vi "HFRR ADV v05.vi"() -> ()   [LabVIEW 2025] (continued)
            n1468 = local write "yflag"(1.0 ("tflag")) -> ()
            n1469 = local write "zflag"(3.0 ("zflag")) -> ()
          }
        }
        n1470 = local read "acq 2"() -> (w2134:bool)
        n1471 = local read "AIR TEMP"() -> (w2097:dbl)
        n1472 = local read "Amb temp"() -> (w2101:dbl)
        n1473 = case shown="True" "Save & Continue" {
          frame False {
          }
          frame True {
            "acq 2" <- TRUE ("acq 2")
          }
        }
        n1474 = case shown="True" "Save & Continue" {
          frame False {
          }
          frame True {
            n1475 = while {
              tunnel: "0123456789abcdefghijklmnopqrstuvwxyzABCDEFGHIJKLMNOPQRSTUVWXYZ" ("string 2") -> [w2294]
              shift-right: [w2292] -> w2287
              shift-left: "" -> [w2291]
              i -> [w2301]
              stop <- w2300 stop-if-true
              n1476 = Random Number (0-1)() -> (number: 0 to 1=w2295:dbl)
              n1477 = Multiply(x=w2295, y=62.0) -> (x*y=w2297:dbl)
              n1478 = Decrement(x="Length") -> (x-1=w2290:i16)
              n1479 = To Word Integer(number=w2297) -> (16bit integer=w2298:i16)
              n1480 = String Subset(string=w2294, offset (0)=w2298, length (rest)=1 ("length (rest)")) -> (substring=w2293:string)
              n1481 = Greater Or Equal?(x=w2301, y=w2290) -> (x >= y?=w2300:bool)
              n1482 = Concatenate Strings(w2293, w2291) -> (w2292:string)
            }
            n1483 = local write "UUID"(w2287) -> ()
          }
        }
        n1484 = case shown="True" "Save & Continue" {
          frame False {
          }
          frame True {
            n1485 = local read "Operator ID"() -> (w2581:string)
            n1486 = local read "FILE"() -> (w2587:string)
            n1487 = String Length(string=w2587) -> (length=w2585:i32)
            n1488 = String Length(string=w2581) -> (length=w2582:i32)
            n1489 = Greater?(x=w2585, y=0) -> (0:w2584:bool)
            n1490 = Greater?(x=w2582, y=0) -> (0:w2580:bool)
            n1491 = And(x=w2584, y=w2580) -> (x .and. y?=w2579:bool)
            n1492 = case shown="True" w2579 {
              frame False {
                n1493 = stacked-sequence {
                  frame #0 {
                    n1494 = One Button Dialog(message="Please Enter a File Name and Operator ID to save data !", button name ("OK")="Ok") -> ()  [unwired: 1 out]
                  }
                  frame #1 {
                    n1495 = local write "Save & Continue"(FALSE ("OK Button")) -> ()
                  }
                }
                n1496 = local write "Save & Continue"(FALSE ("OK Button")) -> ()
              }
              frame True {
                n1497 = stacked-sequence {
                  frame #0 {
                    w2592 = 0.0
                    w2594 = cluster{"y":dbl, dbl, "y":dbl}[] [] ("History Data")
                    w2595 = FALSE ("Heater Button")
                    (unwired) ")!" ("string")
                    (unwired) ")" ("string")
                    w2593 = dbl[] [] ("History Data")
                    w2599 = "\r"
                    # "C:\\WinDucom\\Data\\"
                    # "C:\\LAB-IQ-NXT\\data"
                    n1498 = local write "Humidity ( %RH )"(w2592) -> ()
                    n1499 = local write "Frequency ( Hz )"(w2592) -> ()
                    n1500 = local write "speedop"(0.0 ("PIDclk 2")) -> ()
                    n1501 = local write "Set Temp 2"(w2592) -> ()
                    n1502 = local write "AIR TEMP"(w2592) -> ()
                    n1503 = local write "clk"(0.0 ("clk")) -> ()
                    n1504 = local write "Stroke 4"(w2592) -> ()
                    n1505 = local write "Stroke"(w2592) -> ()
                    n1506 = local write "COF 3"(w2592) -> ()
                    n1507 = local write "COF 2"(w2592) -> ()
                    n1508 = local write "TEMP"(w2592) -> ()
                    n1509 = local write "ecr 3"(w2592) -> ()
                    n1510 = local write "FF 3"(w2592) -> ()
                    n1511 = local write "FF 2"(w2592) -> ()
                    n1512 = property on="Humidity ( %RH )" class="WFChart (strict)"("History Data"=w2593) -> ()  [unwired: 2 in, 2 out]
                    n1513 = property on="Coefficient of Friction" class="WFChart (strict)"("History Data"=w2593) -> ()  [unwired: 2 in, 2 out]
                    n1514 = property on="Coefficient of Friction" class="WFChart (strict)"("History Data"=w2593) -> ()  [unwired: 2 in, 2 out]
                    n1515 = property on="Frictional Force ( N )" class="WFChart (strict)"("History Data"=w2593) -> ()  [unwired: 2 in, 2 out]
                    n1516 = property on="Electrical Contact Resistance ( % )" class="WFChart (strict)"("History Data"=w2593) -> ()  [unwired: 2 in, 2 out]
                    n1517 = property on="Electrical Contact Resistance ( % )" class="WFChart (strict)"("History Data"=w2593) -> ()  [unwired: 2 in, 2 out]
                    n1518 = property on="Temperature ( Deg C )" class="WFChart (strict)"("History Data"=w2593) -> ()  [unwired: 2 in, 2 out]
                    n1519 = property on="Frictional Force ( N )" class="WFChart (strict)"("History Data"=w2593) -> ()  [unwired: 2 in, 2 out]
                    n1520 = property on="Coefficient of Friction" class="WFChart (strict)"("History Data"=w2593) -> ()  [unwired: 2 in, 2 out]
                    n1521 = property on="Frictional Force ( N )" class="WFChart (strict)"("History Data"=w2593) -> ()  [unwired: 2 in, 2 out]
                    n1522 = property on="Electrical Contact Resistance ( % )" class="WFChart (strict)"("History Data"=w2593) -> ()  [unwired: 2 in, 2 out]
                    n1523 = property on="Temperature ( Deg C )" class="WFChart (strict)"("History Data"=w2593) -> ()  [unwired: 2 in, 2 out]
                    n1524 = property on="Humidity ( %RH )" class="WFChart (strict)"("History Data"=w2593) -> ()  [unwired: 2 in, 2 out]
                    n1525 = property on="Stroke ( mm )" class="WFChart (strict)"("History Data"=w2594) -> ()  [unwired: 2 in, 2 out]
                    n1526 = property on="Stroke ( mm )" class="WFChart (strict)"("History Data"=w2594) -> ()  [unwired: 2 in, 2 out]
                    n1527 = local write "Humidity"(w2595) -> ()
                    n1528 = local write "Heater Button"(w2595) -> ()
                    n1529 = local read "NORMAL LOAD"() -> (w2616:dbl)
                    n1530 = Multiply(x=w2616, y=1.0) -> (x*y=w2615:dbl)
                    n1531 = Number To Fractional String(number=w2615, width (-)=i16 5, precision (6)=i16 2) -> (F-format string=w2624:string)  [unwired: 1 in]
                    n1532 = local read "FILE"() -> (w2643:string)
                    n1533 = local read "Fuel Discription :"() -> (w2610:string)
                    n1534 = local read "Batch Ref Num :"() -> (w2597:string)
                    n1535 = Get Date/Time String(date format (0)=enum16{"short", "long", "abbreviated"}."short") -> (date string=w2635:string, time string=w2632:string)  [unwired: 2 in]
                    n1536 = local read "Remarks :"() -> (w2609:string)
                    n1537 = Concatenate Strings("C:\\LAB-IQ-NXT\\data\\" ("string"), w2643) -> (w2642:string)
                    n1538 = Concatenate Strings("Load :- " ("Substring"), w2624, " N ," ("Substring")) -> (w2623:string)
                    n1539 = local read "String 41"() -> (w2601:string)
                    n1540 = Concatenate Strings(w2610) -> (w2611:string)
                    n1541 = Concatenate Strings(w2597) -> (w2596:string)
                    n1542 = Concatenate Strings("tested by") -> (w2605:string)
                    n1543 = Concatenate Strings("(" ("Substring"), w2635, ")" ("Substring"), w2632) -> (w2603:string)
                    "concatenated string" <- w2603
                    n1544 = Concatenate Strings(w2609, "," ("string")) -> (w2608:string)
                    n1545 = Concatenate Strings(w2642, ".duf" ("Substring")) -> (w2639:string)
                    n1546 = Concatenate Strings(w2642, ".dgf" ("Substring")) -> (w2638:string)
                    n1547 = Concatenate Strings("  TIME;      COF;       STROKE;     AIR TEMP;  TEMP;  HUMIDITY;  ECR; PID-OUT; FREQUENCY" ("Substring"), "\r") -> (w2619:string)
                    n1548 = Concatenate Strings(w2601, w2599, "Fuel Discription :-" ("Substring"), w2611, w2599, w2623, w2599, "Batch Ref Num :-" ("Substring"), w2596, w2599, " Remarks :- " ("Substring"), w2608, w2599, " Date :- " ("Substring"), w2603, w2599, "Tested By :-" ("Substring"), w2605) -> (w2617:string)
                    "REMARKS" <- w2617
                    n1549 = String To Path(string=w2638) -> (path=w2636:path)
                    n1550 = String To Path(string=w2639) -> (path=w2613:path)
                    n1551 = call <vilib>:"Write Characters To File.vi"("append to file? (new file:F)"=FALSE, "character string"=w2619, "file path (dialog if empty)"=w2636) -> ()  [unwired: 2 in, 1 out]
                    n1552 = call <vilib>:"Write Characters To File.vi"("append to file? (new file:F)"=FALSE, "character string"=w2617, "file path (dialog if empty)"=w2613) -> ()  [unwired: 2 in, 1 out]
                  }
                  frame #1 {
                    n1553 = local write "Cycles elapsed"(0 ("Cycles elapsed")) -> ()
                    n1554 = local write "cyclecount"(0 ("cyclecount")) -> ()
                    n1555 = local write "Save & Continue"(FALSE ("OK")) -> ()
                    n1556 = local write "autostrtflg"(TRUE ("autostrtflg")) -> ()
                    n1557 = local write "Save"(FALSE ("Save")) -> ()
                    n1558 = Get Date/Time In Seconds() -> (seconds since 1Jan1904=w2648:timestamp)
                    n1559 = To Double Precision Float(number=w2648) -> (double precision float=w2647:dbl)
                    n1560 = local write "acq timer"(w2647) -> ()
                    n1561 = One Button Dialog(message="Please ensure sample is mounted properly and machine is ready in all aspects for testing !", button name ("OK")="Ok") -> ()  [unwired: 1 out]
                  }
                  frame #2 {
                    n1562 = stacked-sequence {
                      frame #0 {
                        n1563 = local write "Main Dashboard Buttons"(T1."Dashboard" ("Main Dashboard Buttons")) -> ()
                        n1564 = local write "Main Tab"(T2."Acquire" ("Main Tab")) -> ()
                      }
                      frame #1 {
                        n1565 = local write "EVENT LOG"("" ("EVENT LOG")) -> ()
                      }
                      frame #2 {
                        n1566 = Wait (ms)(milliseconds to wait=u32 50) -> ()  [unwired: 1 out]
                      }
                      frame #3 {
                        n1567 = local read "EVENT LOG"() -> (w2659:string)
                        n1568 = call "Event Log.vi"("Content"="Test Details", "EVENT LOG"=w2659) -> ("EVENT LOG"=w2658:string)  [unwired: 8 in, 1 out]
                        n1569 = local write "EVENT LOG"(w2658) -> ()
                      }
                      frame #4 {
                        n1570 = Wait (ms)(milliseconds to wait=u32 50) -> ()  [unwired: 1 out]
                      }
                      frame #5 {
                        n1571 = local read "FILE"() -> (w2661:string)
                        n1572 = Concatenate Strings("File Name :" ("Content"), w2661) -> (w2662:string)
                        n1573 = local read "EVENT LOG"() -> (w2665:string)
                        n1574 = call "Event Log.vi"("Content"=w2662, "EVENT LOG"=w2665) -> ("EVENT LOG"=w2664:string)  [unwired: 8 in, 1 out]
                        n1575 = local write "EVENT LOG"(w2664) -> ()
                      }
                      frame #6 {
                        n1576 = Wait (ms)(milliseconds to wait=u32 50) -> ()  [unwired: 1 out]
                      }
                      frame #7 {
                        n1577 = local read "Batch Ref Num :"() -> (w2667:string)
                        n1578 = Concatenate Strings("Batch Ref No :" ("Content"), w2667) -> (w2668:string)
                        n1579 = local read "EVENT LOG"() -> (w2671:string)
                        n1580 = call "Event Log.vi"("Content"=w2668, "EVENT LOG"=w2671) -> ("EVENT LOG"=w2670:string)  [unwired: 8 in, 1 out]
                        n1581 = local write "EVENT LOG"(w2670) -> ()
                      }
                      frame #8 {
                        n1582 = Wait (ms)(milliseconds to wait=u32 50) -> ()  [unwired: 1 out]
                      }
                      frame #9 {
                        n1583 = local read "tested by"() -> (w2673:string)
                        n1584 = Concatenate Strings("Tested By :" ("Content"), w2673) -> (w2674:string)
                        n1585 = local read "EVENT LOG"() -> (w2677:string)
                        n1586 = call "Event Log.vi"("Content"=w2674, "EVENT LOG"=w2677) -> ("EVENT LOG"=w2676:string)  [unwired: 8 in, 1 out]
                        n1587 = local write "EVENT LOG"(w2676) -> ()
                      }
                      frame #10 {
                        n1588 = Wait (ms)(milliseconds to wait=u32 50) -> ()  [unwired: 1 out]
                      }
                      frame #11 {
                        n1589 = local read "TEST STANDARD"() -> (w2680:T3)
                        n1590 = case shown="\"ASTM D6079\", Default" w2680 {
                          tunnel: ["ASTM D6O79" "ISO 12156" "CEC F-096-A-06" "Custom"] -> w2679
                          frame "ASTM D6079", Default {
                          }
                          frame "ISO 12156" {
                          }
                          frame "CEC F-096-A-06" {
                          }
                          frame "Custom" {
                          }
                        }
                        n1591 = Concatenate Strings("Test Standard :" ("Content"), w2679) -> (w2681:string)
                        n1592 = local read "EVENT LOG"() -> (w2684:string)
                        n1593 = call "Event Log.vi"("Content"=w2681, "EVENT LOG"=w2684) -> ("EVENT LOG"=w2683:string)  [unwired: 8 in, 1 out]
                        n1594 = local write "EVENT LOG"(w2683) -> ()
                      }
                      frame #12 {
                        n1595 = Wait (ms)(milliseconds to wait=u32 50) -> ()  [unwired: 1 out]
                      }
                      frame #13 {
                        n1596 = local read "TEST STANDARD"() -> (w2691:T3)
                        n1597 = case shown="\"ASTM D6079\", Default" w2691 {
                          tunnel: ["ASTM D6O79" "ISO 12156" "CEC F-096-A-06" "Custom"] -> w2690
                          frame "ASTM D6079", Default {
                          }
                          frame "ISO 12156" {
                          }
                          frame "CEC F-096-A-06" {
                          }
                          frame "Custom" {
                          }
                        }
                        n1598 = Concatenate Strings("Test Standard :" ("Content"), w2690) -> (w2692:string)
                        n1599 = local read "EVENT LOG"() -> (w2695:string)
                        n1600 = call "Event Log.vi"("Content"=w2692, "EVENT LOG"=w2695) -> ("EVENT LOG"=w2694:string)  [unwired: 8 in, 1 out]
                        n1601 = local write "EVENT LOG"(w2694) -> ()
                      }
                      frame #14 {
                        n1602 = Wait (ms)(milliseconds to wait=u32 50) -> ()  [unwired: 1 out]
                      }
                      frame #15 {
                        n1603 = local read "Fuel Discription :"() -> (w2701:string)
                        n1604 = Concatenate Strings("Fuel Discription :" ("Content"), w2701) -> (w2702:string)
                        n1605 = local read "EVENT LOG"() -> (w2705:string)
                        n1606 = call "Event Log.vi"("Content"=w2702, "EVENT LOG"=w2705) -> ("EVENT LOG"=w2704:string)  [unwired: 8 in, 1 out]
                        n1607 = local write "EVENT LOG"(w2704) -> ()
                      }
                      frame #16 {
                        n1608 = Wait (ms)(milliseconds to wait=u32 50) -> ()  [unwired: 1 out]
                      }
                      frame #17 {
                        n1609 = local read "Remarks :"() -> (w2707:string)
                        n1610 = Concatenate Strings("Remarks :" ("Content"), w2707) -> (w2708:string)
                        n1611 = local read "EVENT LOG"() -> (w2711:string)
                        n1612 = call "Event Log.vi"("Content"=w2708, "EVENT LOG"=w2711) -> ("EVENT LOG"=w2710:string)  [unwired: 8 in, 1 out]
                        n1613 = local write "EVENT LOG"(w2710) -> ()
                      }
                      frame #18 {
                        n1614 = Wait (ms)(milliseconds to wait=u32 50) -> ()  [unwired: 1 out]
                      }
                      frame #19 {
                        n1615 = local read "Operator ID"() -> (w2713:string)
                        n1616 = Concatenate Strings("Operator ID :" ("Content"), w2713) -> (w2715:string)
                        n1617 = local read "EVENT LOG"() -> (w2717:string)
                        n1618 = call "Event Log.vi"("Content"=w2715, "EVENT LOG"=w2717) -> ("EVENT LOG"=w2716:string)  [unwired: 8 in, 1 out]
                        n1619 = local write "EVENT LOG"(w2716) -> ()
                      }
                      frame #20 {
                        n1620 = Wait (ms)(milliseconds to wait=u32 50) -> ()  [unwired: 1 out]
                      }
                      frame #21 {
                        n1621 = local read "EVENT LOG"() -> (w2721:string)
                        n1622 = call "Event Log.vi"("Content"="Test Parameter", "EVENT LOG"=w2721) -> ("EVENT LOG"=w2720:string)  [unwired: 8 in, 1 out]
                        n1623 = local write "EVENT LOG"(w2720) -> ()
                      }
                      frame #22 {
                        n1624 = Wait (ms)(milliseconds to wait=u32 50) -> ()  [unwired: 1 out]
                      }
                      frame #23 {
                        n1625 = local read "Set Hz"() -> (w2725:dbl)
                        n1626 = Number To Fractional String(number=w2725, precision (6)=i16 2) -> (F-format string=w2724:string)  [unwired: 2 in]
                        n1627 = Concatenate Strings("Set Frequency [Hz] :" ("Content"), w2724) -> (w2727:string)
                        n1628 = local read "EVENT LOG"() -> (w2729:string)
                        n1629 = call "Event Log.vi"("Content"=w2727, "EVENT LOG"=w2729) -> ("EVENT LOG"=w2728:string)  [unwired: 8 in, 1 out]
                        n1630 = local write "EVENT LOG"(w2728) -> ()
                      }
                      frame #24 {
                        n1631 = Wait (ms)(milliseconds to wait=u32 50) -> ()  [unwired: 1 out]
                      }
                      frame #25 {
                        n1632 = local read "NORMAL LOAD"() -> (w2732:dbl)
                        n1633 = Number To Fractional String(number=w2732, precision (6)=i16 2) -> (F-format string=w2733:string)  [unwired: 2 in]
                        n1634 = Concatenate Strings("Set Load [N] :" ("Content"), w2733) -> (w2735:string)
                        n1635 = local read "EVENT LOG"() -> (w2737:string)
                        n1636 = call "Event Log.vi"("Content"=w2735, "EVENT LOG"=w2737) -> ("EVENT LOG"=w2736:string)  [unwired: 8 in, 1 out]
                        n1637 = local write "EVENT LOG"(w2736) -> ()
                      }
                      frame #26 {
                        n1638 = Wait (ms)(milliseconds to wait=u32 50) -> ()  [unwired: 1 out]
                      }
                      frame #27 {
                        n1639 = local read "Set Strk"() -> (w2740:dbl)
                        n1640 = Number To Fractional String(number=w2740, precision (6)=i16 2) -> (F-format string=w2741:string)  [unwired: 2 in]
                        n1641 = Concatenate Strings("Set Stroke [mm] :" ("Content"), w2741) -> (w2743:string)
                        n1642 = local read "EVENT LOG"() -> (w2745:string)
                        n1643 = call "Event Log.vi"("Content"=w2743, "EVENT LOG"=w2745) -> ("EVENT LOG"=w2744:string)  [unwired: 8 in, 1 out]
                        n1644 = local write "EVENT LOG"(w2744) -> ()
                      }
                      frame #28 {
                        n1645 = Wait (ms)(milliseconds to wait=u32 50) -> ()  [unwired: 1 out]
                      }
                      frame #29 {
                        n1646 = local read "Set Temp"() -> (w2748:dbl)
                        n1647 = Number To Fractional String(number=w2748, precision (6)=i16 2) -> (F-format string=w2749:string)  [unwired: 2 in]
                        n1648 = Concatenate Strings("Set Temp [deg C] :" ("Content"), w2749) -> (w2751:string)
                        n1649 = local read "EVENT LOG"() -> (w2753:string)
                        n1650 = call "Event Log.vi"("Content"=w2751, "EVENT LOG"=w2753) -> ("EVENT LOG"=w2752:string)  [unwired: 8 in, 1 out]
                        n1651 = local write "EVENT LOG"(w2752) -> ()
                      }
                      frame #30 {
                        n1652 = Wait (ms)(milliseconds to wait=u32 50) -> ()  [unwired: 1 out]
                      }
                      frame #31 {
                        n1653 = local read "Set Rh"() -> (w2756:dbl)
                        n1654 = Number To Fractional String(number=w2756, precision (6)=i16 2) -> (F-format string=w2757:string)  [unwired: 2 in]
                        n1655 = Concatenate Strings("Set Humidity [%RH] :" ("Content"), w2757) -> (w2759:string)
                        n1656 = local read "EVENT LOG"() -> (w2761:string)
                        n1657 = call "Event Log.vi"("Content"=w2759, "EVENT LOG"=w2761) -> ("EVENT LOG"=w2760:string)  [unwired: 8 in, 1 out]
                        n1658 = local write "EVENT LOG"(w2760) -> ()
                      }
                      frame #32 {
                        n1659 = Wait (ms)(milliseconds to wait=u32 50) -> ()  [unwired: 1 out]
                      }
                      frame #33 {
                        n1660 = local read "test time"() -> (w2764:dbl)
                        n1661 = Number To Fractional String(number=w2764, precision (6)=i16 1) -> (F-format string=w2765:string)  [unwired: 2 in]
                        n1662 = Concatenate Strings("Test Time [mins] :" ("Content"), w2765) -> (w2767:string)
                        n1663 = local read "EVENT LOG"() -> (w2769:string)
                        n1664 = call "Event Log.vi"("Content"=w2767, "EVENT LOG"=w2769) -> ("EVENT LOG"=w2768:string)  [unwired: 8 in, 1 out]
                        n1665 = local write "EVENT LOG"(w2768) -> ()
                      }
                    }
                  }
                }
              }
            }
          }
        }
        n1666 = local read "Set Rh"() -> (w2103:dbl)
        n1667 = Add(x=w2104, y=w2129) -> (x+y=w2130:dbl)
        n1668 = Subtract(x=w2104, y=w2129) -> (x-y=w2131:dbl)
        n1669 = Add(x=w2102, y=w2123) -> (x+y=w2124:dbl)
        n1670 = Subtract(x=w2102, y=w2123) -> (x-y=w2125:dbl)
        n1671 = And(x=w2134, y=w2135) -> (x .and. y?=w2133:bool)
        n1672 = Greater Or Equal?(x=w2097, y=15.0) -> (x >= y?=w2098:bool)
        "powstat" <- w2098
        n1673 = local read "Humidity ( %RH )"() -> (w2100:dbl)
        n1674 = case shown="True" w2133 {
          frame False {
            n1675 = local write "tfalg"(0.0 ("tfalg")) -> ()
          }
          frame True {
            n1676 = local read "tfalg"() -> (w2278:dbl)
            n1677 = Equal?(x=w2278, y=0.0) -> (x = y?=w2279:bool)
            n1678 = case shown="True" w2279 {
              frame False {
              }
              frame True {
                n1679 = local read "Total No. of Tests"() -> (w2282:dbl)
                n1680 = local write "tfalg"(1.0 ("tfalg")) -> ()
                n1681 = local write "acq 2"(FALSE ("acq 2")) -> ()
                n1682 = Wait (ms)(milliseconds to wait=u32 200) -> ()  [unwired: 1 out]
                n1683 = Increment(x=w2282) -> (x+1=w2281:dbl)
                n1684 = local write "Total No. of Tests"(w2281) -> ()
              }
            }
          }
        }
        n1685 = In Range and Coerce(upper limit=w2130, x=w2101, lower limit=w2131) -> (In Range?=w2120:bool)  [unwired: 1 out]
        n1686 = Add(x=w2103, y=w2128) -> (x+y=w2127:dbl)
        n1687 = Subtract(x=w2103, y=w2128) -> (x-y=w2126:dbl)
        n1688 = local read "TEMP"() -> (w2099:dbl)
        n1689 = local write "Test \nStatus"(w2139) -> ()
        n1690 = local write "st enable"(w2139) -> ()
        n1691 = local write "PWR"(w2139) -> ()
        n1692 = local write "Save"(w2139) -> ()
        n1693 = local read "Main Tab"() -> (w2096:T2)
        n1694 = case shown="True" w2120 {
          tunnel: [FALSE ("RUN") TRUE ("RUN")] -> w2119
          tunnel: [_ 1] -> w2112
          frame False {
          }
          frame True {
          }
        }
        n1695 = In Range and Coerce(upper limit=w2127, x=w2100, lower limit=w2126) -> (In Range?=w2118:bool)  [unwired: 1 out]
        n1696 = In Range and Coerce(upper limit=w2124, x=w2099, lower limit=w2125) -> (In Range?=w2116:bool)  [unwired: 1 out]
        n1697 = case shown="True" w2132 {
          frame False {
            n1698 = local read "Rt 3"() -> (w2260:bool)
            n1699 = case shown="True" w2260 {
              frame False {
              }
              frame True {
                n1700 = local write "Rt 3"(FALSE ("Rt 3")) -> ()
                n1701 = local write "Json End Flg"(TRUE ("Upld AR 2")) -> ()
              }
            }
            "Rt" <- TRUE ("Rt")
            "Rt 2" <- FALSE ("Rt")
          }
          frame True {
            n1702 = local read "Rt"() -> (w2267:bool)
            n1703 = local write "Rt 2"(TRUE ("Rt 2")) -> ()
            n1704 = case shown="True" w2267 {
              frame False {
              }
              frame True {
                w2268 = TRUE ("Upld AR 2")
                n1705 = local write "Rt"(FALSE ("Rt")) -> ()
                n1706 = local write "Upld AR"(w2268) -> ()
                n1707 = local write "Json St Flg"(w2268) -> ()
              }
            }
            "Rt 3" <- TRUE ("Rt 3")
          }
        }
        n1708 = case shown="True" w2118 {
          tunnel: [FALSE ("RUN") TRUE ("RUN")] -> w2117
          tunnel: [_ 2] -> w2111
          frame False {
          }
          frame True {
          }
        }
        n1709 = case shown="True" w2116 {
          tunnel: [FALSE ("RUN") TRUE ("RUN")] -> w2115
          tunnel: [_ 3] -> w2110
          frame False {
          }
          frame True {
          }
        }
        n1710 = case shown="\"Acquire\"" w2096 {
          tunnel: w2098 -> [_ w2329]
          frame Default {
            w2328 = 0.0 ("output")
            n1711 = local write "PID-out"(w2328) -> ()
            n1712 = local write "Frequency ( Hz )"(w2328) -> ()
          }
          frame "Acquire" {
            n1713 = stacked-sequence {
              frame #0 {
                n1714 = local read "clk"() -> (w2349:dbl)
                n1715 = local read "Save"() -> (w2345:bool)
                n1716 = Equal?(x=w2349, y=0.0) -> (x = y?=w2346:bool)
                n1717 = case shown="True" "RUN" {
                  tunnel: [w2354 w2362] -> w2332
                  frame False {
                    w2354 = 0.0
                    n1718 = local write "Reinit PID"(TRUE) -> ()
                    n1719 = property on="Stroke" class="DigNum (strict)"("Visible"=TRUE) -> ()  [unwired: 2 in, 2 out]
                    n1720 = property on="Stroke 2" class="DigNum (strict)"("Visible"=FALSE) -> ()  [unwired: 2 in, 2 out]
                    n1721 = local write "String 14"("Test will autostart once parameters reach the set value." ("String 14")) -> ()
                    n1722 = local write "Old Pid Val"(w2354) -> ()
                  }
                  frame True {
                    n1723 = property on="Stroke 2" class="DigNum (strict)"("Visible"=TRUE) -> ()  [unwired: 2 in, 2 out]
                    n1724 = property on="Stroke" class="DigNum (strict)"("Visible"=FALSE) -> ()  [unwired: 2 in, 2 out]
                    n1725 = property on="STOP 2" class="Bool (strict)"("Disabled"=u8 2) -> ()  [unwired: 2 in, 2 out]
                    n1726 = property on="RUN" class="Bool (strict)"("Visible"=TRUE) -> ()  [unwired: 2 in, 2 out]
                    n1727 = local read "PID Ref"() -> (w2373:bool)
                    n1728 = case shown="True" w2373 {
                      tunnel: [w2374 w2390] -> w2372
                      frame False {
                        n1729 = local read "Old Pid Val"() -> (w2374:dbl)
                      }
                      frame True {
                        n1730 = local read "Set Hz"() -> (w2383:dbl)
                        n1731 = local read "Frequency"() -> (w2394:dbl)
                        n1732 = Add(x=w2383, y=10.0) -> (x+y=w2392:dbl)
                        n1733 = Add(x=w2383, y=-10.0 ("Offset")) -> (x+y=w2401:dbl)
                        n1734 = Add(x=w2383, y=-10.0) -> (x+y=w2393:dbl)
                        n1735 = In Range and Coerce(upper limit=w2392, x=w2394, lower limit=w2393) -> (coerced(x)=w2382:dbl)  [unwired: 1 out]
                        n1736 = Or(x="Reinit PID", y="Reinit PID") -> (x .or. y?=w2391:bool)
                        n1737 = Multiply(x=w2401, y=0.1 ("Gain")) -> (x*y=w2380:dbl)
                        n1738 = local read "Elapsed time"() -> (w2387:dbl)
                        n1739 = local read "SPEED OUT:"() -> (w2402:dbl)
                        n1740 = Add(x=w2380, y=1.5) -> (x+y=w2378:dbl)
                        n1741 = call-poly <vilib>:"PID.vi"("reinitialize? (F)"=w2391, "output range"=cluster{"output high":dbl, "output low":dbl} {"output high"=1.0, "output low"=-1.0}, "PID gains"=T10 {"proportional gain (Kc)"=0.0005, "integral time (Ti, min)"=0.001, "derivative time (Td, min)"=0.0} ("Motor PID"), "process variable"=w2382, "setpoint"=w2383) -> ("output"=w2381:dbl)  [unwired: 5 in, 1 out]
                        n1742 = Multiply(x=w2378, y=w2402) -> (x*y=w2377:dbl)
                        n1743 = Greater?(x=w2387, y=0.05) -> (0:w2386:bool)
                        n1744 = case shown="True" w2386 {
                          tunnel: w2381 -> [_ w2404]
                          tunnel: [0.0 ("output") w2404] -> w2384
                          frame False {
                          }
                          frame True {
                            n1745 = local write "Reinit PID"(FALSE ("Reinit PID")) -> ()
                          }
                        }
                        n1746 = Multiply(x=w2377, y=0.8) -> (x*y=w2376:dbl)
                        n1747 = Add(x=w2376, y=w2384) -> (x+y=w2389:dbl)
                        n1748 = flat-sequence {
                          tunnel: [w2407] -> w2390
                          tunnel: w2389 -> [w2407]
                          frame #0 {
                            n1749 = local write "PID Ref"(FALSE ("PID Ref")) -> ()
                          }
                        }
                      }
                    }
                    "Old Pid Val" <- w2372
                    n1750 = local write "String 14"(" Running....." ("String 14")) -> ()
                    n1751 = local read "Set Hz"() -> (w2369:dbl)
                    n1752 = call <vilib>:"Uniform White Noise Waveform.vi"() -> ("signal out"=w2368:waveform(dbl))  [unwired: 10 in, 1 out]
                    n1753 = local read "Freq"() -> (w2361:dbl)
                    n1754 = Add(x=w2369, y=w2368) -> (x+y=w2367:waveform(dbl))
                    n1755 = Multiply(x=w2367, y=ext 0.1) -> (x*y=w2363:waveform(ext))
                    n1756 = Multiply(x=w2361, y=0.9) -> (x*y=w2364:dbl)
                    n1757 = Add(x=w2363, y=w2364) -> (x+y=w2362:waveform(ext))
                  }
                }
                n1758 = And(x=w2346, y=w2345) -> (x .and. y?=w2347:bool)
                n1759 = Not(x="Engage") -> (.not. x?=w2336:bool)
                n1760 = case shown="True" w2347 {
                  frame False {
                  }
                  frame True {
                    n1761 = local write "clk"(10.0 ("clk")) -> ()
                    n1762 = Get Date/Time In Seconds() -> (seconds since 1Jan1904=w2410:timestamp)
                    n1763 = To Double Precision Float(number=w2410) -> (double precision float=w2408:dbl)
                    n1764 = local write "acq timer"(w2408) -> ()
                    n1765 = local write "act save time"(w2408) -> ()
                  }
                }
                n1766 = call "Elapsed Time"("Time Target (s)"="Countdown", "Reset"=w2336) -> ("Elapsed Time (s)"=w2341:dbl, "Time has Elapsed"=w2339:bool)  [unwired: 10 in, 6 out]
                "Countdown 2" <- w2341
                n1767 = Subtract(x=w2341, y=2.0) -> (x-y=w2344:dbl)
                n1768 = Less?(x=w2344, y="Countdown") -> (x < y?=w2342:bool)
                n1769 = And(x=w2342, y=w2339) -> (x .and. y?=w2338:bool)
                n1770 = case shown="True" w2338 {
                  frame False {
                  }
                  frame True {
                    (unwired) dbl[] [] ("History Data")
                    n1771 = local write "Engage"(FALSE ("Engage")) -> ()
                    n1772 = local write "RUN"(TRUE ("RUN")) -> ()
                    n1773 = local read "Humidity ( %RH )"() -> (→"Rh Before":dbl)
                  }
                }
                n1774 = local read "Test \nStatus"() -> (w2334:bool)
                n1775 = Select(t=w2332, s=w2334, f=0.0) -> (s? t:f=w2333:dbl)
                n1776 = local write "Frequency ( Hz )"(w2333) -> ()
                n1777 = local write "Freq"(w2333) -> ()
              }
              frame #1 {
                w2433 = 1000000.0 ("x")
                # "Elapsed time\ncof\nstroke\nAir temp\nTemp\nHumidity"
                # "acq timer\n\nact save time"
                # "convert to microseconds"
                n1778 = local read "COUNT"() -> (w2416:i32)
                n1779 = local read "Rate"() -> (w2429:dbl)
                n1780 = Divide(x=w2433, y=w2429) -> (x/y=w2434:dbl)
                n1781 = Greater Or Equal?(x=w2416, y=250) -> (x >= y?=w2415:bool)
                n1782 = Get Date/Time In Seconds() -> (seconds since 1Jan1904=w2436:timestamp)
                n1783 = case shown="True" w2415 {
                  frame False {
                    n1784 = local read "COUNT"() -> (w2437:i32)
                    n1785 = Increment(x=w2437) -> (x+1=w2438:i32)
                    n1786 = local write "COUNT"(w2438) -> ()
                  }
                  frame True {
                    n1787 = local write "COUNT"(0 ("COUNT")) -> ()
                  }
                }
                n1788 = local read "Samplingtime 2"() -> (w2414:dbl)
                n1789 = local read "act save time"() -> (w2431:dbl)
                n1790 = Divide(x=w2434, y=w2433) -> (x/y=w2432:dbl)
                n1791 = To Double Precision Float(number=w2436) -> (double precision float=w2425:dbl)
                n1792 = Add(x=w2431, y=w2414) -> (x+y=w2430:dbl)
                n1793 = local read "acq timer"() -> (w2435:dbl)
                n1794 = local read "COUNT"() -> (w2418:i32)
                n1795 = Greater Or Equal?(x=w2425, y=w2430) -> (x >= y?=w2413:bool)
                n1796 = Multiply(x=w2432, y=w2418) -> (x*y=w2424:dbl)
                n1797 = Subtract(x=w2425, y=w2435) -> (x-y=w2427:dbl)
                n1798 = local read "Save"() -> (w2428:bool)
                n1799 = Add(x=w2427, y=w2424) -> (x+y=w2411:dbl)
                "Elapsed time 3" <- w2411
                n1800 = And(x=w2413, y=w2428) -> (x .and. y?=w2426:bool)
                n1801 = case shown="True" w2426 {
                  tunnel: w2425 -> [_ w2521]
                  tunnel: [FALSE ("Boolean 2") TRUE ("Boolean 2")] -> _
                  frame False {
                  }
                  frame True {
                    w2467 = ";" ("Substring")
                    # "Pid out/\nFreq response value"
                    n1802 = local write "act save time"(w2521) -> ()
                    n1803 = local read "Set Strk"() -> (w2491:dbl)
                    n1804 = local read "Stroke"() -> (w2482:dbl)
                    n1805 = local read "FF 2"() -> (w2478:dbl)
                    "Frictional Force ( N )" <- w2478
                    "Frictional Force ( N )" <- w2478
                    n1806 = local write "FF 3"(w2478) -> ()
                    n1807 = Subtract(x=w2482, y=w2491) -> (x-y=w2488:dbl)
                    n1808 = local read "COF 2"() -> (w2473:dbl)
                    "cof" <- w2473
                    "Coefficient of Friction" <- w2473
                    "COF 4" <- w2473
                    "Coefficient of Friction" <- w2473
                    n1809 = local write "COF 3"(w2473) -> ()
                    n1810 = Multiply(x=w2488, y=0.05) -> (x*y=w2490:dbl)
                    n1811 = local read "TEMP"() -> (w2477:dbl)
                    "Temp" <- w2477
                    "Temperature ( Deg C )" <- w2477
                    n1812 = Add(x=w2490, y=w2491) -> (x+y=w2471:dbl)
                    "Stroke Ln" <- w2471
                    "Disp" <- w2471
                    n1813 = local read "ecr"() -> (w2474:dbl)
                    "ecr 2" <- w2474
                    "Electrical Contact Resistance ( % )" <- w2474
                    "ecr 4" <- w2474
                    n1814 = local read "Humidity ( %RH )"() -> (w2476:dbl)
                    "Humidity ( %RH )" <- w2476
                    "Humidity ( %RH )" <- w2476
                    n1815 = local read "Frequency ( Hz )"() -> (w2484:dbl)
                    n1816 = local read "Elapsed time"() -> (w2514:dbl)
                    n1817 = local read "AIR TEMP"() -> (w2481:dbl)
                    n1818 = local write "ecr 3"(w2474) -> ()
                    n1819 = local read "PID-out"() -> (w2487:dbl)
                    n1820 = local write "Temperature ( Deg C )"(w2477) -> ()
                    n1821 = local write "Electrical Contact Resistance ( % )"(w2474) -> ()
                    n1822 = local read "FILE"() -> (w2522:string)
                    n1823 = Number To Fractional String(number=w2471, width (-)=i16 9 ("precision (6)"), precision (6)=i16 6) -> (F-format string=w2507:string)  [unwired: 1 in]
                    n1824 = Number To Fractional String(number=w2481, width (-)=i16 9 ("precision (6)"), precision (6)=i16 3) -> (F-format string=w2506:string)  [unwired: 1 in]
                    n1825 = Number To Fractional String(number=w2477, width (-)=i16 9 ("precision (6)"), precision (6)=i16 3) -> (F-format string=w2503:string)  [unwired: 1 in]
                    n1826 = Number To Fractional String(number=w2476, width (-)=i16 9 ("precision (6)"), precision (6)=i16 3) -> (F-format string=w2500:string)  [unwired: 1 in]
                    n1827 = Number To Fractional String(number=w2474, width (-)=i16 9 ("precision (6)"), precision (6)=i16 3) -> (F-format string=w2496:string)  [unwired: 1 in]
                    n1828 = Number To Fractional String(number=w2487, width (-)=i16 9 ("precision (6)"), precision (6)=i16 3) -> (F-format string=w2492:string)  [unwired: 1 in]
                    n1829 = Number To Fractional String(number=w2484, width (-)=i16 9 ("precision (6)"), precision (6)=i16 3) -> (F-format string=w2483:string)  [unwired: 1 in]
                    n1830 = Number To Fractional String(number=w2473, width (-)=i16 9 ("precision (6)"), precision (6)=i16 6) -> (F-format string=w2515:string)  [unwired: 1 in]
                    n1831 = Number To Fractional String(number=w2514, width (-)=i16 14 ("precision (6)"), precision (6)=i16 3) -> (F-format string=w2516:string)  [unwired: 1 in]
                    n1832 = Bundle("y"=1.02, w2471, "y"=0.08) -> (w2475:cluster{"y":dbl, dbl, "y":dbl})  [unwired: 1 in]
                    n1833 = Number To Fractional String(number="Ambient Humidity :", width (-)=i16 9 ("precision (6)"), precision (6)=i16 6) -> (F-format string=w2465:string)  [unwired: 1 in]
                    n1834 = local read "RUN"() -> (w2472:bool)
                    n1835 = Concatenate Strings("C:\\LAB-IQ-NXT\\Data\\" ("string"), w2522, ".dgf" ("Substring")) -> (w2524:string)
                    n1836 = case shown="True" w2472 {
                      tunnel: w2475 -> [_ w2530]
                      tunnel: w2471 -> [_ w2529]
                      tunnel: w2471 -> [_ w2528]
                      tunnel: w2471 -> [_ w2527]
                      frame False {
                      }
                      frame True {
                        "Stroke ( mm )" <- w2530
                        "Stroke ( mm )" <- w2530
                        "Stroke 4" <- w2529
                        "Stroke 3" <- w2528
                        "Stroke 2" <- w2527
                      }
                    }
                    n1837 = String To Path(string=w2524) -> (path=w2523:path)
                    n1838 = Concatenate Strings(w2516, w2467, w2515, w2467, w2507, w2467, w2506, w2467, w2503, w2467, w2500, w2467, w2496, w2467, w2492, w2467, w2483, w2467, w2465, "\r") -> (w2513:string)
                    n1839 = call <vilib>:"Write Characters To File.vi"("append to file? (new file:F)"=TRUE, "character string"=w2513, "file path (dialog if empty)"=w2523) -> ()  [unwired: 2 in, 1 out]
                    "refresh flag" <- TRUE ("refresh flag")
                  }
                }
                n1840 = Divide(x=w2411, y=60.0) -> (x/y=w2422:dbl)
                n1841 = local read "Test \nStatus"() -> (w2412:bool)
                n1842 = local read "clk"() -> (w2419:dbl)
                n1843 = Equal?(x=w2419, y=10.0) -> (x = y?=w2421:bool)
                n1844 = case shown="True" w2412 {
                  tunnel: w2422 -> [_ w2445]
                  tunnel: w2427 -> [_ w2456]
                  tunnel: [0.0 w2452] -> _
                  tunnel: w2421 -> [_ w2451]
                  tunnel: [0.0 w2450] -> _
                  tunnel: w2411 -> [_ w2450]
                  tunnel: w2425 -> [w2441 _]
                  frame False {
                    n1845 = local write "acq timer"(w2441) -> ()
                    n1846 = local write "Test Duration Status"(0.0 ("Test Duration Status")) -> ()
                  }
                  frame True {
                    n1847 = local read "Set Hz"() -> (w2453:dbl)
                    n1848 = local write "Elapsed time"(w2445) -> ()
                    n1849 = local read "test time"() -> (w2444:dbl)
                    n1850 = Multiply(x=w2456, y=w2453) -> (x*y=w2455:dbl)
                    n1851 = case shown="False" w2451 {
                      tunnel: w2455 -> [w2457 _]
                      tunnel: [w2457 1.0] -> w2452
                      frame False {
                        n1852 = local write "Cycles elapsed"(w2457) -> ()
                      }
                      frame True {
                      }
                    }
                    n1853 = Greater?(x=w2445, y=w2444) -> (0:w2454:bool)
                    n1854 = Subtract(x=w2444, y=w2445) -> (x-y=w2449:dbl)
                    "time" <- w2449
                    n1855 = case shown="True" w2454 {
                      frame False {
                      }
                      frame True {
                        n1856 = local write "RUN"(FALSE ("OK Button 2")) -> ()
                        n1857 = property on="STOP 2" class="Bool (strict)"("Disabled"=u8 0) -> ()  [unwired: 2 in, 2 out]
                        n1858 = local read "Humidity ( %RH )"() -> (→"Rh After":dbl)
                        n1859 = local write "Heater Button"(FALSE ("Heater Button")) -> ()
                        n1860 = local write "Humidity"(FALSE ("Humidity")) -> ()
                      }
                    }
                    n1861 = local write "Time Remaining"(w2449) -> ()
                    n1862 = Divide(x=w2445, y=w2444) -> (x/y=w2448:dbl)
                    n1863 = Multiply(x=w2448, y=100.0) -> (x*y=w2446:dbl)
                    n1864 = local write "Test Duration Status"(w2446) -> ()
                  }
                }
              }
              frame #2 {
                n1865 = case shown="True" "Heater Button" {
                  tunnel: [0.0 ("output") w2552] -> w2531
                  frame False {
                    w2533 = TRUE ("tmpchk")
                    n1866 = local read "TEMP"() -> (w2534:dbl)
                    n1867 = local write "Temp ini"(w2534) -> ()
                    n1868 = local write "Reset 4"(w2533) -> ()
                    n1869 = local write "tmpchk"(w2533) -> ()
                    n1870 = local write "reinit"(TRUE ("reinit")) -> ()
                  }
                  frame True {
                    # "Logic to turn off\nthe heater when \ntemp is not rising.\nTime - 60 sec\nDelta t- 5°c"
                    n1871 = local read "Temp ini"() -> (w2540:dbl)
                    n1872 = Less?(x=w2540, y=53.0) -> (x < y?=w2538:bool)
                    n1873 = And(x="tmpchk", y=w2538) -> (x .and. y?=w2541:bool)
                    n1874 = case shown="True" w2541 {
                      frame False {
                      }
                      frame True {
                        n1875 = call "Elapsed Time8"("Time Target (s)"=300.0, "Reset"="Reset 4") -> ("Time has Elapsed"=w2557:bool)  [unwired: 10 in, 7 out]
                        n1876 = flat-sequence {
                          tunnel: w2557 -> [_]
                          frame #0 {
                            n1877 = local write "Reset 4"(FALSE ("Reset 4")) -> ()
                          }
                        }
                        n1878 = case shown="True" w2557 {
                          frame False {
                          }
                          frame True {
                            n1879 = local read "Temp ini"() -> (w2564:dbl)
                            n1880 = Add(x=w2564, y=5.0) -> (x+y=w2562:dbl)
                            n1881 = local read "TEMP"() -> (w2565:dbl)
                            n1882 = Greater?(x=w2565, y=w2562) -> (0:w2563:bool)
                            n1883 = case shown="False" w2563 {
                              frame False {
                                n1884 = local write "Heater Button"(FALSE ("Heater Button")) -> ()
                              }
                              frame True {
                                n1885 = local write "tmpchk"(FALSE ("tmpchk")) -> ()
                              }
                            }
                          }
                        }
                      }
                    }
                    n1886 = local read "Set Temp"() -> (w2549:dbl)
                    n1887 = local read "TEMP"() -> (w2543:dbl)
                    n1888 = call-poly <vilib>:"PID.vi"("reinitialize? (F)"="reinit", "output range"="output range", "dt (s)"=-1.0, "PID gains"="Temp PID gains", "process variable"=w2543, "setpoint"=w2549) -> ("output"=w2546:dbl)  [unwired: 4 in, 1 out]
                    n1889 = Subtract(x=w2549, y=w2543) -> (x-y=w2551:dbl)
                    n1890 = Add(x=w2549, y=0.5) -> (x+y=w2547:dbl)
                    n1891 = Greater Or Equal?(x=w2543, y=w2547) -> ()  [unwired: 1 out]
                    n1892 = Select(t=0.0, s=FALSE, f=w2546) -> (s? t:f=w2545:dbl)
                    "PID output" <- w2545
                    n1893 = flat-sequence {
                      tunnel: w2545 -> [w2568]
                      tunnel: [w2568] -> w2552
                      frame #0 {
                        n1894 = local write "reinit"(FALSE ("reinit")) -> ()
                      }
                    }
                    n1895 = Bundle(w2551, "output"=w2545, "TEMP"=w2543) -> (→"gTEMP 3":cluster{dbl, "output":dbl, "TEMP":dbl})  [unwired: 1 in]
                  }
                }
                "PID-out" <- w2531
              }
              frame #3 {
                n1896 = local read "TEMP"() -> (w2570:dbl)
                n1897 = Greater Or Equal?(x=w2570, y="Set Temp 2") -> (x >= y?=w2575:bool)
                n1898 = case shown="True" w2575 {
                  tunnel: [FALSE TRUE] -> w2573
                  frame False {
                  }
                  frame True {
                  }
                }
                "Status 13" <- w2573
                n1899 = And(x=w2573, y="trip1 8") -> (x .and. y?=w2572:bool)
                n1900 = case shown="True" w2572 {
                  frame False {
                  }
                  frame True {
                    w2576 = FALSE ("OK Button 2")
                    n1901 = local write "RUN"(w2576) -> ()
                    n1902 = local write "Heater Button"(w2576) -> ()
                  }
                }
              }
            }
            n1903 = case shown="False" w2329 {
              frame False {
                n1904 = stacked-sequence {
                  frame #0 {
                    n1905 = local write "RUN"(FALSE ("OK Button 2")) -> ()
                  }
                  frame #1 {
                  }
                }
              }
              frame True {
              }
            }
          }
        }
        n1906 = local read "airtempflg"() -> (w2121:bool)
        n1907 = Or(x=w2121, y=w2119) -> (x .or. y?=w2122:bool)
        n1908 = Insert Into Array(array=string[] ["Air Temperature has reached set value,", "Humidity has reached set value,", "Sample Temperaturehas reached set value,", ""], index=0, new element="") -> (w2107:string[])
        n1909 = disable-structure shown="Disabled" {
          disable-tunnel: w2122 -> [w2199 _]
          disable-tunnel: w2117 -> [w2198 _]
          disable-tunnel: w2115 -> [w2197 _]
          frame Disabled {
            n1910 = Compound Arithmetic op=AND(w2199, w2198, w2197) -> ()  [unwired: 1 out]
            n1911 = case shown="True" {
              selector: _ -> [_ _]
              frame False {
              }
              frame True {
                w2200 = FALSE ("autostrtflg")
                n1912 = local write "RUN"(TRUE ("RUN")) -> ()
                n1913 = local write "autostrtflg"(w2200) -> ()
                n1914 = local write "autostart"(w2200) -> ()
                n1915 = local write "String 14"(" Running....." ("String 14")) -> ()
              }
            }
          }
          frame Enabled {
          }
        }
        n1916 = Build Array(w2112, w2111, w2110) -> (w2108:i32[])
        n1917 = for {
          tunnel: w2108 -> [w2250] mode=indexing
          tunnel: w2107 -> [w2249]
          shift-right: [w2246] -> w2106
          shift-left: "" -> [w2248]
          n1918 = Index Array(array=w2249, index=w2250) -> (element=w2247:string)
          n1919 = Concatenate Strings(w2247, w2248) -> (w2246:string)
        }
        n1920 = local write "autostart 2"(w2106) -> ()
        n1921 = local read "Reset Graph"() -> (w2095:bool)
        n1922 = case shown="True" w2095 {
          selector: w2095 -> [_ w2149]
          frame False {
          }
          frame True {
            w2163 = 0.0 ("X Scale.Range:Maximum")
            n1923 = Not(x=w2149) -> (.not. x?=w2148:bool)
            n1924 = local write "Reset Graph"(w2148) -> ()
            n1925 = property on="Electrical Contact Resistance ( % )" class="WFChart (strict)"("XScale.Maximum"=600.0 ("X Scale.Range:Maximum"), "XScale.Minimum"=0.0 ("X Scale.Range:Minimum"), "YScale.Maximum"=100.0 ("Y Scale.Range:Maximum"), "YScale.Minimum"=0.0 ("Y Scale.Range:Minimum")) -> ()  [unwired: 2 in, 2 out]
            n1926 = property on="Frictional Force ( N )" class="WFChart (strict)"("XScale.Maximum"=600.0 ("X Scale.Range:Maximum"), "XScale.Minimum"=0.0 ("X Scale.Range:Minimum"), "YScale.Maximum"=100.0 ("Y Scale.Range:Maximum"), "YScale.Minimum"=0.0 ("Y Scale.Range:Minimum")) -> ()  [unwired: 2 in, 2 out]
            n1927 = property on="Temperature ( Deg C )" class="WFChart (strict)"("XScale.Maximum"=600.0 ("X Scale.Range:Maximum"), "XScale.Minimum"=0.0 ("X Scale.Range:Minimum"), "YScale.Maximum"=100.0 ("Y Scale.Range:Maximum"), "YScale.Minimum"=0.0 ("Y Scale.Range:Minimum")) -> ()  [unwired: 2 in, 2 out]
            n1928 = property on="Humidity ( %RH )" class="WFChart (strict)"("XScale.Maximum"=600.0 ("X Scale.Range:Maximum"), "XScale.Minimum"=0.0 ("X Scale.Range:Minimum"), "YScale.Maximum"=100.0 ("Y Scale.Range:Maximum"), "YScale.Minimum"=0.0 ("Y Scale.Range:Minimum")) -> ()  [unwired: 2 in, 2 out]
            n1929 = property on="Stroke ( mm )" class="WFChart (strict)"("XScale.Maximum"=600.0 ("X Scale.Range:Maximum"), "XScale.Minimum"=0.0 ("X Scale.Range:Minimum"), "YScale.Maximum"=100.0 ("Y Scale.Range:Maximum"), "YScale.Minimum"=0.0 ("Y Scale.Range:Minimum")) -> ()  [unwired: 2 in, 2 out]
            n1930 = property on="Coefficient of Friction" class="WFChart (strict)"("XScale.Maximum"=600.0 ("X Scale.Range:Maximum"), "XScale.Minimum"=0.0 ("X Scale.Range:Minimum"), "YScale.Maximum"=100.0 ("Y Scale.Range:Maximum"), "YScale.Minimum"=0.0 ("Y Scale.Range:Minimum")) -> ()  [unwired: 2 in, 2 out]
            n1931 = property on="Electrical Contact Resistance ( % )" class="WFChart (strict)"("XScale.Minimum"=0.0 ("X Scale.Range:Minimum"), "XScale.Maximum"=600.0 ("X Scale.Range:Maximum"), "YScale.Minimum"=0.0 ("Y Scale.Range:Minimum"), "YScale.Maximum"=100.0 ("Y Scale.Range:Maximum")) -> ()  [unwired: 2 in, 2 out]
            n1932 = property on="Temperature ( Deg C )" class="WFChart (strict)"("XScale.Minimum"=0.0 ("X Scale.Range:Minimum"), "XScale.Maximum"=600.0 ("X Scale.Range:Maximum"), "YScale.Minimum"=0.0 ("Y Scale.Range:Minimum"), "YScale.Maximum"=100.0 ("Y Scale.Range:Maximum")) -> ()  [unwired: 2 in, 2 out]
            n1933 = property on="Coefficient of Friction" class="WFChart (strict)"("XScale.Minimum"=0.0 ("X Scale.Range:Minimum"), "XScale.Maximum"=600.0 ("X Scale.Range:Maximum"), "YScale.Maximum"=1.0 ("X Scale.Range:Minimum"), "YScale.Minimum"=0.0 ("X Scale.Range:Minimum")) -> ()  [unwired: 2 in, 2 out]
            n1934 = property on="Frictional Force ( N )" class="WFChart (strict)"("XScale.Maximum"=600.0 ("X Scale.Range:Maximum"), "XScale.Minimum"=w2163, "YScale.Maximum"=10.0 ("Y Scale.Range:Maximum"), "YScale.Minimum"=w2163) -> ()  [unwired: 2 in, 2 out]
            n1935 = property on="Stroke ( mm )" class="WFChart (strict)"("XScale.Maximum"=600.0 ("X Scale.Range:Maximum"), "XScale.Minimum"=0.0 ("X Scale.Range:Minimum"), "YScale.Maximum"=100.0 ("Y Scale.Range:Maximum"), "YScale.Minimum"=0.0 ("Y Scale.Range:Minimum")) -> ()  [unwired: 2 in, 2 out]
            n1936 = property on="Humidity ( %RH )" class="WFChart (strict)"("XScale.Maximum"=600.0 ("X Scale.Range:Maximum"), "XScale.Minimum"=0.0 ("X Scale.Range:Minimum"), "YScale.Maximum"=100.0 ("Y Scale.Range:Maximum"), "YScale.Minimum"=0.0 ("Y Scale.Range:Minimum")) -> ()  [unwired: 2 in, 2 out]
          }
        }
      }
      frame "Compare Files" {
        # "Elapsed time\ncof\nstroke\nAir temp\nTemp\nHumidity"
        n1937 = case shown="True" "RSTV1 2" {
          frame False {
          }
          frame True {
            n1938 = property on="Humidity" class="XYGraph (strict)"("Y Scale.Display Format:Precision"=u8 0 ("Y Scale.Format & Precision:Precision")) -> ()  [unwired: 2 in, 2 out]
            n1939 = property on="Humidity" class="XYGraph (strict)"("X Scale.Range:Minimum"=0.0, "X Scale.Range:Maximum"=75.0, "Y Scale.Range:Minimum"=48.0, "Y Scale.Range:Maximum"=58.0) -> ()  [unwired: 2 in, 2 out]
          }
        }
        n1940 = case shown="True" "RST CP 2" {
          frame False {
          }
          frame True {
